vi "Curtin_BuildConfigInfo.vi"(10 "Test Template in":string, 11 "ComboBox in":refnum<vi>) -> (2 "String":string, 3 "template":string)   [LabVIEW 2022 SP3]
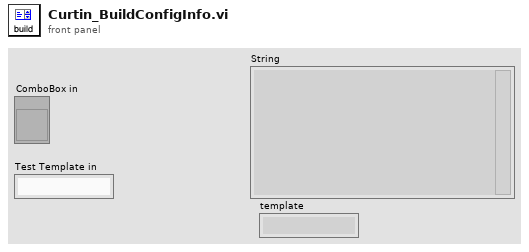
[diagram p1: front panel]
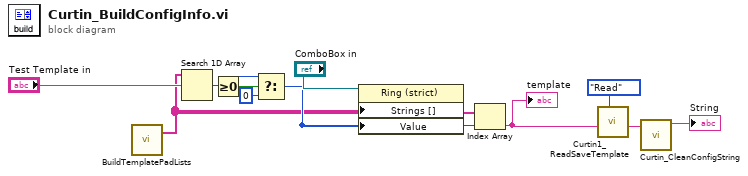
[diagram p0: block diagram]
diagram:
  n1 = call "BuildTemplatePadLists.vi"() -> ("All Templates"=w1:string[])  [unwired: 8 in, 3 out]
  n2 = Search 1D Array(1D array=w1, element="Test Template in") -> (index of element=w7:i32)  [unwired: 1 in]
  n3 = Greater Or Equal To 0?(x=w7) -> (x >= 0?=w10:bool)
  n4 = Select(t=w7, s=w10, f=0) -> (s? t:f=w6:i32)
  n5 = property on="Property Node" class="Ring (strict)"(reference="ComboBox in", "Strings []"=w1, "Value"=w6) -> ()  [unwired: 1 in, 2 out]
  n6 = Index Array(array=w1, index=w6) -> (element=w3:string)
  "template" <- w3
  n7 = call "Curtin1_ReadSaveTemplate.vi"("Task"=enum16{"Save", "Read", "List"}."Read", "Template"=w3) -> ("String"=w2:string)  [unwired: 6 in, 3 out]
  n8 = call "Curtin_CleanConfigString.vi"("String in"=w2) -> ("String out"=→"String":string)  [unwired: 10 in]
